vi "Main_08B.vi"() -> ()   [LabVIEW 2024]
uses:
  Map_Antena.ctl
  Cluster_Position.ctl
  <vilib>/Utility/miscctls.llb/LVMapReplaceAction.ctl
panel:
  out "final":string[][](array[string])
  out "Antena Map":T1
  out "2D Array":string[][](array[string])
  in  "Use Puzzle":bool
  out "Answer":u32
  in  "Puzzle":string="............s...............1.....................\n......................E......3.....S..............\n.......................3.....S....................\n...e........T.t.......S.1...........I.............\n..................B..................I.....O......\ng.......z........i39......B..I....................\n.......s....S.......3......................i..I...\n....e.............2..........B....................\n.......tC...z.......g......1......................\n.E......s....R....................................\n..G...t..........2................................\n.........K...C.......2............................\n....T..e...........5...C..........................\n...T................................O...o.........\n...............................g..............o...\n.........z...................g......i............o\n...9.E............H...........Y.......O...........\n..........R..H...............7.O..................\n...........H.............v......7........B........\n..9.Q.......................W......1........Y.....\n.........................z.7.................Y....\n.....Q................................v...........\n....K.......E.....R...............2..........o....\n.n............H......v...........................Y\n.G.y..........................Q...................\n......G....A5.....................h...............\n..........D...5.w...9.............................\n......n....5...L..................................\n............................v.....................\n............L...0t..........7.....................\n..n....k............y....................W........\n..k..........0.........................W..........\n...n.......R..L..a........................W.......\n.........................................h........\n..0..L........c...b...............................\n.....................8.y..........................\n.......w.................6.............h.......N..\n..........y..4....................................\n...0....8...k.....Z........r......................\n..............a...8Z.........G......4.............\n........4..b.q.....................K..............\n.q...........kZ.K......b..D.........d.............\n.8.....................D................r.........\n.....w.........a...............d........A.........\n................................d.A.hV............\n................c..........D.....V....r...........\n.......Z......6.....l........................A.d..\n...................l..6..c....b......r...........N\n......a....4........q..l..V..c................N...\nl.....w...........q..6............V..............."
  in  "Example":string="............\n........0...\n.....0......\n.......0....\n....0.......\n......A.....\n............\n............\n........A...\n.........A..\n............\n............"
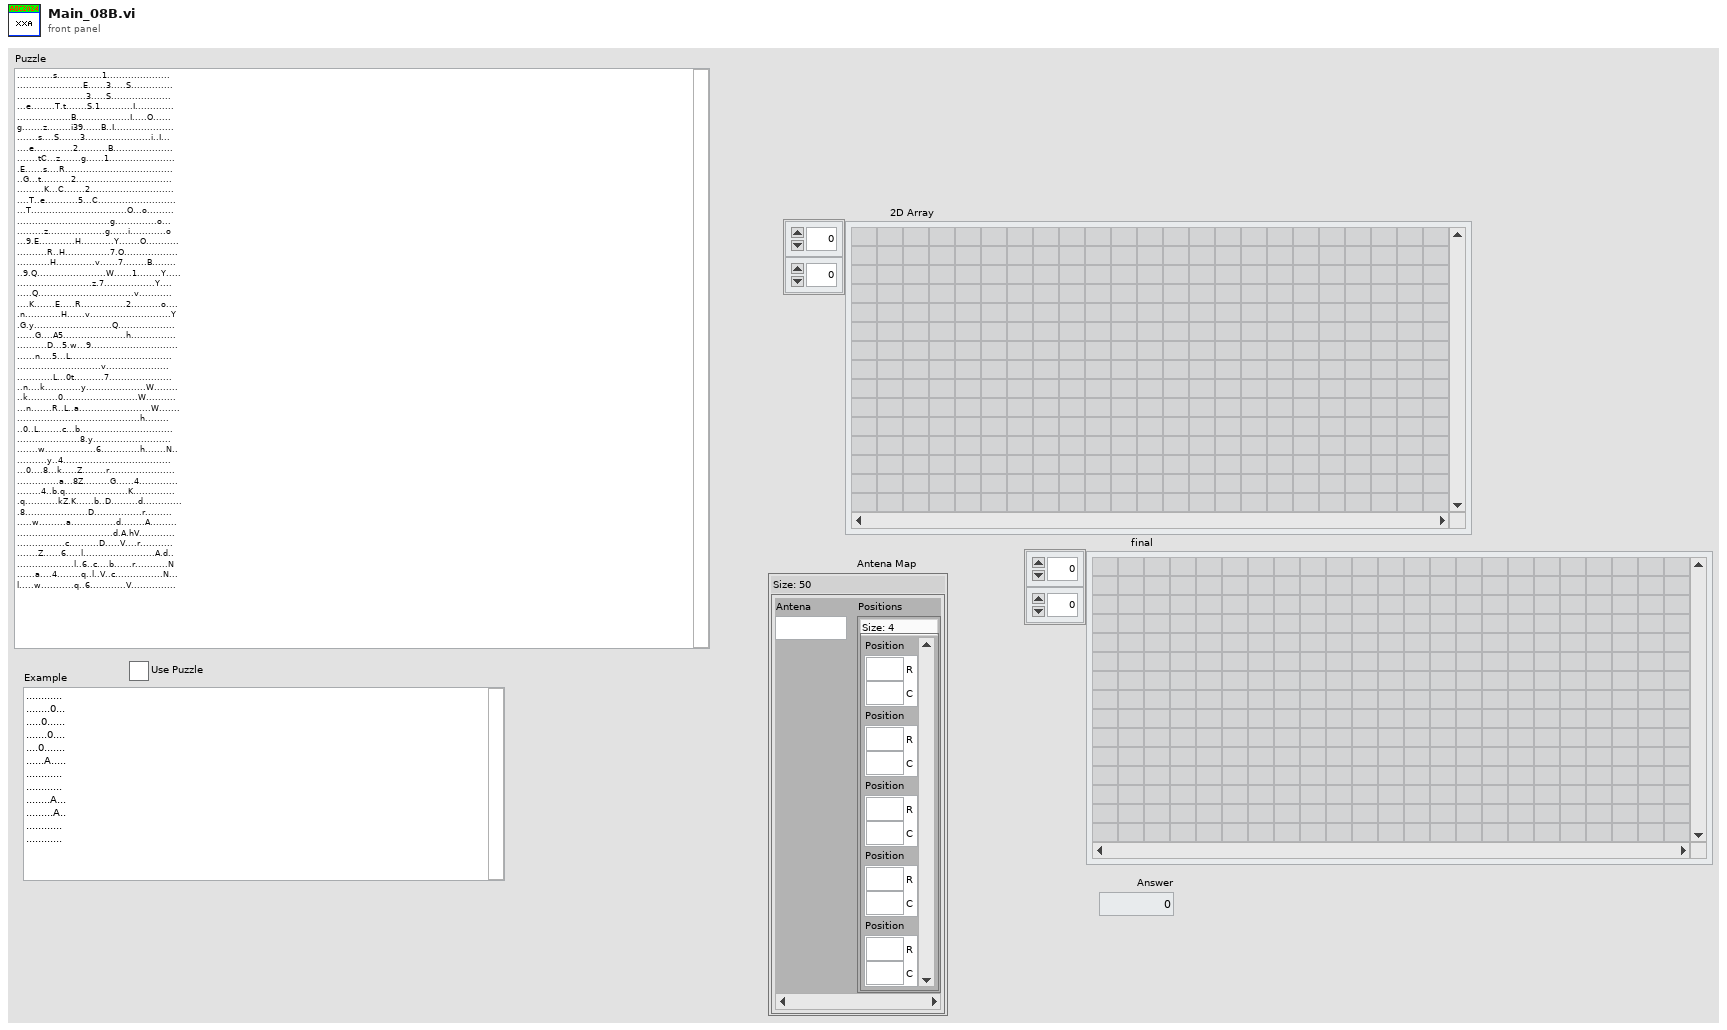
[diagram p1: front panel]
types:
  T1 = typedef "Map_Antena.ctl" = map{string, set{T2}}
  T2 = typedef "Cluster_Position.ctl" = cluster{"R":i32, "C":i32}
  T3 = typedef "LVMapReplaceAction.ctl" = enum32{"Modify Entry only if found", "Add or Modify Entry", "Delete Entry"}
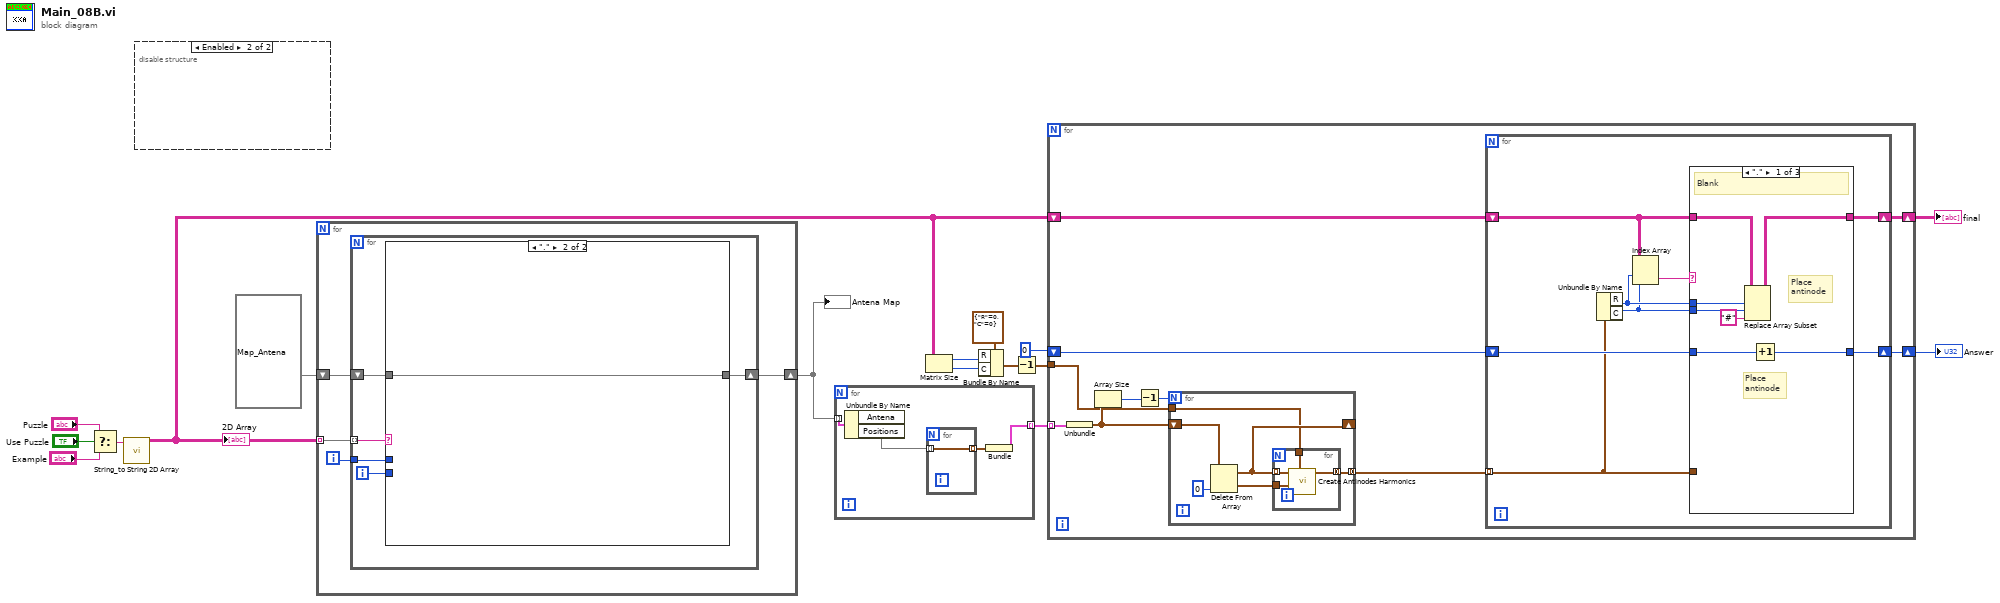
[diagram p0: block diagram]
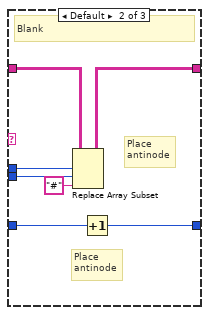
[diagram p2: hidden frame]
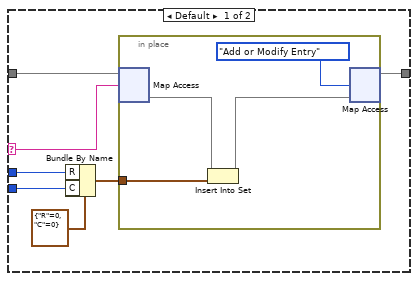
[diagram p4: hidden frame]
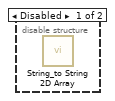
[diagram p5: hidden frame]
diagram:
  n1 = Select(t="Puzzle", s="Use Puzzle", f="Example") -> (s? t:f=w13:string)
  n2 = call "String_to String 2D Array.vi"("Input String"=w13) -> ("2D Array"=w4:string[][])  [unwired: 10 in]
  "2D Array" <- w4
  n3 = disable-structure shown="Enabled" {
    frame Disabled {
      n4 = call "String_to String 2D Array.vi"() -> ()  [unwired: 11 in, 1 out]
    }
    frame Enabled {
    }
  }
  n5 = for {
    tunnel: w4 -> [w20] mode=indexing
    shift-right: [w18] -> w11
    shift-left: T1 {} ("Antena Map") -> [w19]
    i -> [w17]
    n6 = for {
      tunnel: w20 -> [w25] mode=indexing
      shift-right: [w21] -> w18
      shift-left: w19 -> [w24]
      tunnel: w17 -> [w23]
      i -> [w22]
      n7 = case shown="\".\"" w25 {
        selector: w25 -> [w31 _]
        tunnel: w24 -> [w32 w37]
        tunnel: w23 -> [w29 _]
        tunnel: w22 -> [w28 _]
        tunnel: [w26 w37] -> w21
        frame Default {
          n8 = Bundle By Name(cluster=T2 {"R"=0, "C"=0} ("Position"), "R"=w29, "C"=w28) -> (w27:T2)
          n9 = in-place {
            in-place-border: w27 -> [w33]
            n10 = in-place-map #1(w32, w31) -> (w35:set{T2})  [unwired: 1 in, 1 out]
            n11 = Insert Into Set(10:w33, 11:w35) -> (3:w34:set{T2})  [unwired: 1 out]
            n12 = in-place-map #1(w34, LVMapReplaceAction."Add or Modify Entry" ("action")) -> (w26:T1)  [unwired: 2 out]
          }
        }
        frame "." {
        }
      }
    }
  }
  "Antena Map" <- w11
  n13 = for {
    tunnel: w11 -> [w41] mode=indexing
    tunnel: [w38] -> w10 mode=indexing
    n14 = Unbundle By Name(w41) -> ("Positions"=w40:set{T2})  [unwired: 1 out]
    n15 = for {
      tunnel: w40 -> [w42] mode=indexing
      tunnel: [w42] -> w39 mode=indexing
    }
    n16 = Bundle(w39) -> (w38:cluster{T2[]})  [unwired: 1 in]
  }
  n17 = Matrix Size(0:w4) -> (1:w8:i32, 2:w7:i32)
  n18 = Bundle By Name(cluster=T2 {"R"=0, "C"=0} ("Position"), "R"=w8, "C"=w7) -> (w6:T2)
  n19 = Decrement(x=w6) -> (x-1=w5:T2)
  n20 = for {
    tunnel: w10 -> [w52] mode=indexing
    tunnel: w5 -> [w44]
    shift-right: [w46] -> w2
    shift-left: u32 0 -> [w47]
    shift-right: [w45] -> w1
    shift-left: w4 -> [w48]
    n21 = Unbundle(w52) -> (w51:T2[])
    n22 = Array Size(array=w51) -> (size(s)=w50:i32)
    n23 = Decrement(x=w50) -> (x-1=w49:i32)
    n24 = for {
      N: w49 -> [_]
      shift-right: [w79] -> _
      shift-left: w51 -> [w82]
      tunnel: [w78] -> w43 mode=concatenating
      tunnel: w44 -> [w77]
      n25 = Delete From Array(array=w82, index=0) -> (deleted portion=w80:T2, array with subset deleted=w79:T2[])  [unwired: 1 in]
      n26 = for {
        tunnel: w80 -> [w85]
        tunnel: w79 -> [w86] mode=indexing
        tunnel: [w83] -> w78 mode=concatenating
        tunnel: w77 -> [w84]
        n27 = call "Create Antinodes Harmonics.vi"("Max Grid Index"=w84, "Antena 2"=w85, "Antena 1"=w86) -> ("Antinodes"=w83:T2[])  [unwired: 8 in]
      }
    }
    n28 = for {
      shift-right: [w59] -> w45
      shift-left: w48 -> [w60]
      shift-right: [w57] -> w46
      shift-left: w47 -> [w58]
      tunnel: w43 -> [w53] mode=indexing
      n29 = Unbundle By Name(w53) -> ("R"=w55:i32, "C"=w54:i32)
      n30 = Index Array(array=w60, index (row)=w55, index (col)=w54) -> (element=w56:string)
      n31 = case shown="\".\"" w56 {
        tunnel: w60 -> [w67 w74 w76]
        tunnel: w53 -> [_ _ _]
        tunnel: w55 -> [w65 w72 _]
        tunnel: w54 -> [w64 w71 _]
        tunnel: [w66 w73 w76] -> w59
        tunnel: w58 -> [w62 w69 w75]
        tunnel: [w61 w68 w75] -> w57
        frame "." {
          # "Place\nantinode"
          # "Place\nantinode"
          # "Blank"
          n32 = Replace Array Subset(array=w67, new element="#" ("new element/subarray"), index (row)=w65, index (col)=w64) -> (w66:string[][])
          n33 = Increment(x=w62) -> (x+1=w61:u32)
        }
        frame Default {
          # "Place\nantinode"
          # "Place\nantinode"
          # "Blank"
          n34 = Replace Array Subset(array=w74, new element="#" ("new element/subarray"), index (row)=w72, index (col)=w71) -> (w73:string[][])
          n35 = Increment(x=w69) -> (x+1=w68:u32)
        }
        frame "#" {
        }
      }
    }
  }
  "Answer" <- w2
  "final" <- w1
